vi "OE1022_Configure Channel Out.vi"(7 "OE1022_Configure Channel Out":T1={"CH1"=0, "CH2"=0, "Speed"=0, "CH2 Offset(%)"=0.0, "CH1 Offset(%)"=0.0, "CH2 Expand"=1, "CH1 Expand"=1} {"CH1 Expand" min=1 max=256; "CH2 Expand" min=1 max=256; "CH1 Offset(%)" min=-100.0 max=100.0 format="%#.2g"; "CH2 Offset(%)" min=-100.0 max=100.0 format="%#.2g"; "Speed" items=["Slow", "Fast"]; "CH2" items=["R", "X", "Y", "Theta", "Rh1", "Xh1", "Yh1", "Theta h1", "Rh2", "Xh2", "Yh2", "Theta h2", "Noise", "E1", "E2", "E3", "E4"]; "CH1" items=["R", "X", "Y", "Theta", "Rh1", "Xh1", "Yh1", "Theta h1", "Rh2", "Xh2", "Yh2", "Theta h2", "Noise", "E1", "E2", "E3", "E4"]}, 8 "Error in (no error)":errorcluster caption="error out（no error）", 9 "Remote Mode":u16(ring) items=["USB"=0, "GPIB"=2], 11 "VISA resource name":refnum<visa-resource-name>) -> (0 "Error out":errorcluster caption="error out", 1 "Output String":string, 3 "VISA resource  out":refnum<visa-resource-name>)   [LabVIEW 2011]
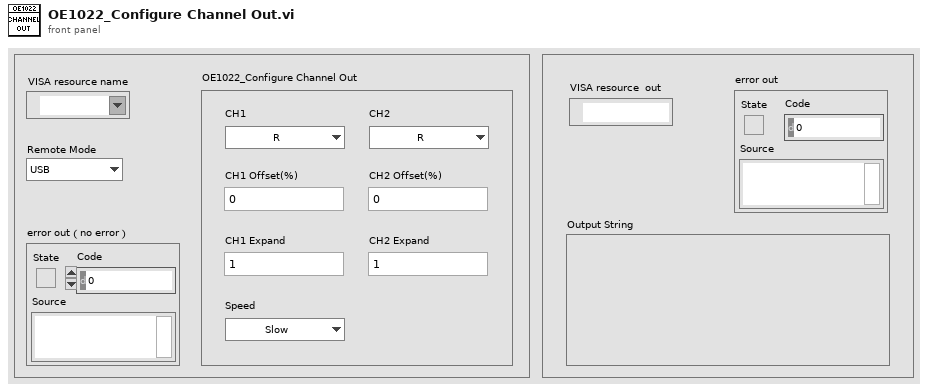
[diagram p1: front panel]
types:
  T1 = cluster{"CH1":u16, "CH2":u16, "Speed":u16, "CH2 Offset(%)":dbl, "CH1 Offset(%)":dbl, "CH2 Expand":i16, "CH1 Expand":i16}
  T2 = enum16{"ISRC", "IGND", "ICPL", "ILIN", "PHAS", "FMOD", "RSLP", "FREQ", "SWPT", "SLLM", "SULM", "SSLL", "SSLG", "STLM", "SWRM", "IRNG", "SENS", "RMOD", "OFLT", "OFSL", "SYNC", "DMOD", "HARM", "DARB", "SWVT", "SLVL", "SVLL", "SVUL", "SVSL", "SVSG", "SVTM", "SVRM", "RALL", "SNAP", "OUTP", "OAUX", "COUT", "CAUX", "COFP", "CEXP", "FPOP", "OEXP", "*IDN", "*RST", "OVLD", "INOV", "GNOV", "*PLL", "SSET", "RSET", "AGAN", "APHS", "ARSV", "ASCL", "EQCD", "EQCS", "SPED", "SRAT", "SLEN", "SSLE", "STRG", "SPRM", "STRD", "PAUS", "REST", "SPTS", "TRCA", "TEMP", "RSTU", "IHNZ", "DEQU", "SADD", "ARNG", "CSPE", "ISRCD", "IGNDD", "ICPLD", "ILIND", "PHASD", "FMODD", "RSLPD", "FREQD", "SWPTD", "SLLMD", "SULMD", "SSLLD", "SSLGD", "STLMD", "SWRMD", "SENSD", "RMODD", "OFLTD", "OFSLD", "SYNCD", "HARMD", "EQCDD", "EQCSD", "SNAPD", "OUTPD", "SWVTD", "SLVLD", "SVLLD", "SVULD", "SVSLD", "SVSGD", "SVTMD", "SVRMD", "SVDCD", "ARSVD", "AGAND", "APHSD", "ASCLD", "FPOPD", "CAUXD", "OEXPD", "SPEDD", "SRATD", "SLEND", "SSLED", "STRGD", "SPRMD", "STRDD", "PAUSD", "RESTD", "SPTSD", "TRCAD", "*IDND", "*RSTD", "INOVD", "GNOVD", "*PLLD", "SSETD", "RSETD"}
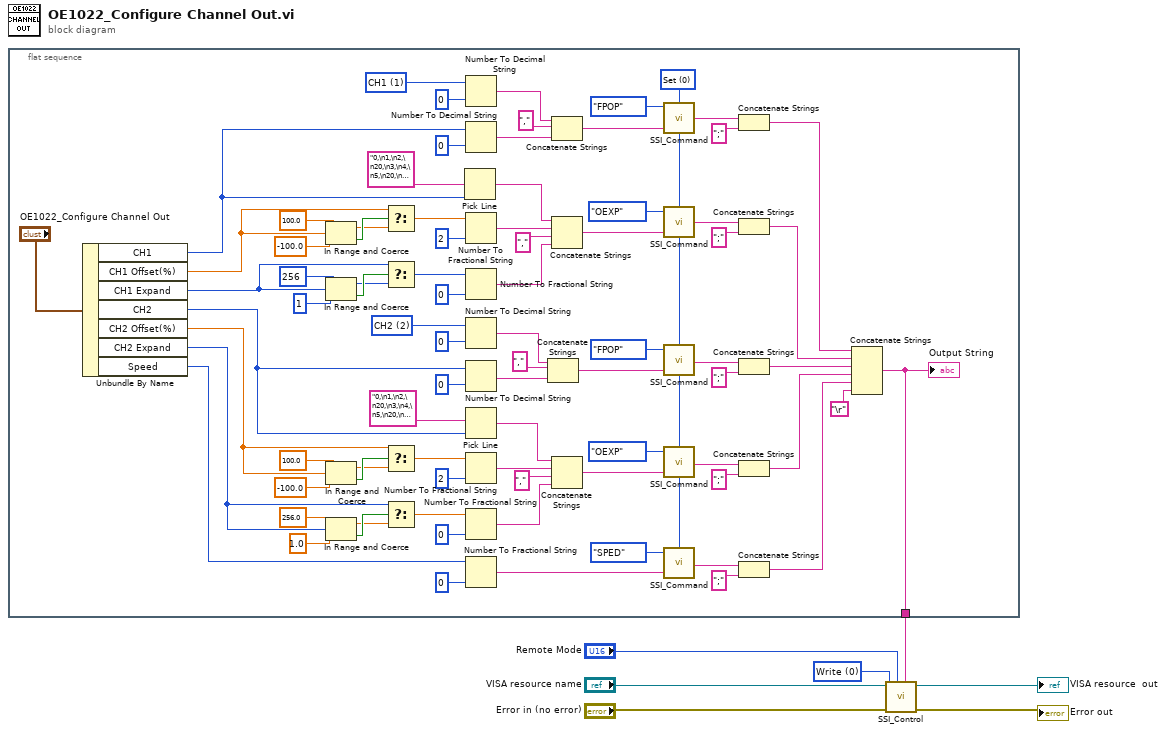
[diagram p0: block diagram]
diagram:
  w6 = u16 0 items=["Write", "Read"] ("Control")
  n1 = flat-sequence {
    tunnel: [w74] -> w1
    frame #0 {
      w42 = u16 2 items=["CH1"=1, "CH2"=2]
      w41 = u16 1 items=["CH1"=1, "CH2"=2]
      w20 = u16 0 items=["Set", "Query"] ("Opera")
      n2 = Unbundle By Name("OE1022_Configure Channel Out") -> ("CH1"=w12:u16, "CH1 Offset(%)"=w49:dbl, "CH1 Expand"=w50:i16, "CH2"=w8:u16, "CH2 Offset(%)"=w52:dbl, "CH2 Expand"=w51:i16, "Speed"=w16:u16)
      n3 = In Range and Coerce(upper limit=100.0 ("上限"), x=w49, lower limit=-100.0 ("下限")) -> (coerced(x)=w57:dbl, In Range?=w58:bool)
      n4 = In Range and Coerce(upper limit=u16 256 ("上限"), x=w50, lower limit=u16 1 ("下限")) -> (coerced(x)=w14:u16, In Range?=w68:bool)
      n5 = In Range and Coerce(upper limit=100.0 ("上限"), x=w52, lower limit=-100.0 ("下限")) -> (coerced(x)=w84:dbl, In Range?=w85:bool)
      n6 = In Range and Coerce(upper limit=256.0 ("上限"), x=w51, lower limit=1.0 ("下限")) -> (coerced(x)=w62:dbl, In Range?=w63:bool)
      n7 = Select(t=w49, s=w58, f=w57) -> (s? t:f=w27:dbl)
      n8 = Select(t=w50, s=w68, f=w14) -> (s? t:f=w64:u16)
      n9 = Select(t=w52, s=w85, f=w84) -> (s? t:f=w65:dbl)
      n10 = Select(t=w51, s=w63, f=w62) -> (s? t:f=w59:dbl)
      n11 = Pick Line(multi-line string="0,\n1,\n2,\n20,\n3,\n4,\n5,\n20,\n6,\n7,\n8,\n20,\n9,\n20,\n20,\n20,\n20," ("多行字符串"), line index=w12) -> (output string=w11:string)  [unwired: 1 in]
      n12 = Number To Decimal String(number=w41, width (-)=i16 0 ("精度(6)")) -> (decimal integer string=w39:string)
      n13 = Number To Decimal String(number=w12, width (-)=i16 0 ("精度(6)")) -> (decimal integer string=w24:string)
      n14 = Number To Fractional String(number=w27, precision (6)=i16 2 ("精度(6)")) -> (F-format string=w38:string)  [unwired: 2 in]
      n15 = Number To Fractional String(number=w64, precision (6)=i16 0 ("精度(6)")) -> (F-format string=w37:string)  [unwired: 2 in]
      n16 = Number To Decimal String(number=w42, width (-)=i16 0 ("精度(6)")) -> (decimal integer string=w36:string)
      n17 = Number To Decimal String(number=w8, width (-)=i16 0 ("精度(6)")) -> (decimal integer string=w25:string)
      n18 = Pick Line(multi-line string="0,\n1,\n2,\n20,\n3,\n4,\n5,\n20,\n6,\n7,\n8,\n20,\n9,\n20,\n20,\n20,\n20," ("多行字符串"), line index=w8) -> (output string=w10:string)  [unwired: 1 in]
      n19 = Number To Fractional String(number=w65, precision (6)=i16 2 ("精度(6)")) -> (F-format string=w35:string)  [unwired: 2 in]
      n20 = Number To Fractional String(number=w59, precision (6)=i16 0 ("精度(6)")) -> (F-format string=w34:string)  [unwired: 2 in]
      n21 = Number To Fractional String(number=w16, precision (6)=i16 0 ("精度(6)")) -> (F-format string=w17:string)  [unwired: 2 in]
      n22 = Concatenate Strings(w36, ",", w25) -> (w32:string)
      n23 = Concatenate Strings(w39, ",", w24) -> (w40:string)
      n24 = Concatenate Strings(w11, w38, ",", w37) -> (w31:string)
      n25 = Concatenate Strings(w10, w35, ",", w34) -> (w33:string)
      n26 = call "SSI_Command.vi"("Opera"=w20, "Paramter"=w40, "Command Type"=T2."FPOP") -> ("Output string"=w76:string)  [unwired: 1 in]
      n27 = call "SSI_Command.vi"("Opera"=w20, "Paramter"=w31, "Command Type"=T2."OEXP") -> ("Output string"=w80:string)  [unwired: 1 in]
      n28 = call "SSI_Command.vi"("Opera"=w20, "Paramter"=w32, "Command Type"=T2."FPOP") -> ("Output string"=w78:string)  [unwired: 1 in]
      n29 = call "SSI_Command.vi"("Opera"=w20, "Paramter"=w33, "Command Type"=T2."OEXP") -> ("Output string"=w69:string)  [unwired: 1 in]
      n30 = call "SSI_Command.vi"("Opera"=w20, "Paramter"=w17, "Command Type"=T2."SPED") -> ("Output string"=w21:string)  [unwired: 1 in]
      n31 = Concatenate Strings(w76, ";" ("替换字符串(\"\")")) -> (w48:string)
      n32 = Concatenate Strings(w80, ";" ("替换字符串(\"\")")) -> (w47:string)
      n33 = Concatenate Strings(w78, ";" ("替换字符串(\"\")")) -> (w46:string)
      n34 = Concatenate Strings(w69, ";" ("替换字符串(\"\")")) -> (w45:string)
      n35 = Concatenate Strings(w21, ";" ("替换字符串(\"\")")) -> (w19:string)
      n36 = Concatenate Strings(w48, w47, w46, w45, w19, "\r") -> (w74:string)
      "Output String" <- w74
    }
  }
  n37 = call "SSI_Control.vi"("Write Buffer"=w1, "Remote Mode"="Remote Mode", "Error in (no error)"="Error in (no error)", "Control"=w6, "VISA resource name"="VISA resource name") -> ("Error out"=→"Error out":errorcluster, "VISA resource  out"=→"VISA resource  out":refnum<visa-resource-name>)  [unwired: 3 in, 2 out]
